vi "Save-Recall Cal Kit.vi"(0 "VISA resource name":refnum<visa-resource-name>, 1 "saver's name":string, 2 "saved cal kit comments":string, 5 "save/load":bool, 7 "file name (read description)":path, 11 "error in (no error)":errorcluster, 12 "saved cal kit title":string) -> (3 "recaller's name":string, 4 "VISA resource name out":refnum<visa-resource-name>, 6 "recalled cal kit comments":string, 8 "recalled cal kit date":string, 10 "recalled cal kit time":string, 14 "recalled cal kit title":string, 15 "error out":errorcluster)   [LabVIEW 2018, in "Agilent 87XX Series.lvlib"]
doc: "This VI for the HP8753B Network Analyzer is used to save and recall modified calibration kit information. The cal kit information is encoded as a form 1 string."
uses:
  Agilent 87XX Series.lvlib
panel:
  # "save to file\nrecall from file"
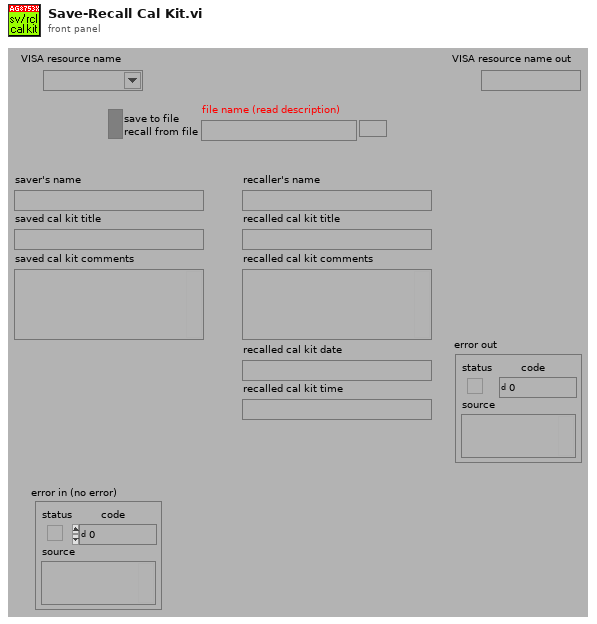
[diagram p1: front panel]
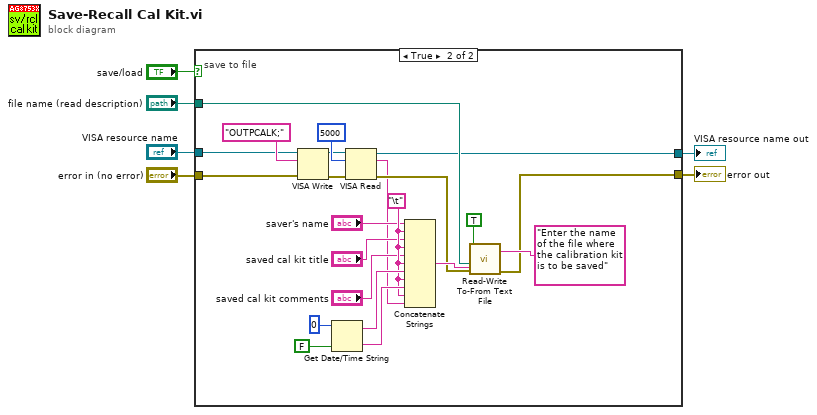
[diagram p0: block diagram]
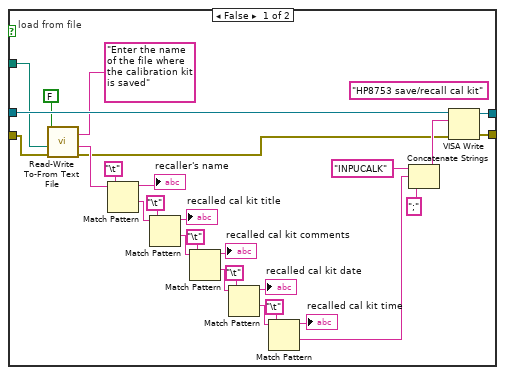
[diagram p2: hidden frame]
diagram:
  n1 = case shown="True" "save/load" {
    tunnel: "file name (read description)" -> [w15 w44]
    tunnel: "VISA resource name" -> [w16 w45]
    tunnel: "error in (no error)" -> [w9 w40]
    tunnel: [w11 w37] -> w2
    tunnel: [w10 w38] -> w1
    frame False {
      (unwired) "HP8753 save/recall cal kit"
      # "load from file"
      n2 = call "Read-Write To-From Text File.vi"("dialog box prompt"="Enter the name of the file where the calibration kit is saved", "error in (no error)"=w9, "file name (read description)"=w15, "read/write (f:read)"=FALSE) -> ("error out"=w8:errorcluster, "string which was read"=w13:string)  [unwired: 6 in]
      n3 = Match Pattern(string=w13, regular expression="\t") -> (before substring=→"recaller's name":string, after substring=w28:string)  [unwired: 1 in, 2 out]
      n4 = Match Pattern(string=w28, regular expression="\t") -> (before substring=→"recalled cal kit title":string, after substring=w27:string)  [unwired: 1 in, 2 out]
      n5 = Match Pattern(string=w27, regular expression="\t") -> (before substring=→"recalled cal kit comments":string, after substring=w23:string)  [unwired: 1 in, 2 out]
      n6 = Match Pattern(string=w23, regular expression="\t") -> (before substring=→"recalled cal kit date":string, after substring=w26:string)  [unwired: 1 in, 2 out]
      n7 = Match Pattern(string=w26, regular expression="\t") -> (before substring=→"recalled cal kit time":string, after substring=w7:string)  [unwired: 1 in, 2 out]
      n8 = Concatenate Strings("INPUCALK", w7, ";") -> (w32:string)
      n9 = VISA Write(VISA resource name=w16, write buffer=w32, error in (no error)=w8) -> (VISA resource name out=w11:refnum<visa-resource-name>, error out=w10:errorcluster)  [unwired: 1 out]
    }
    frame True {
      w49 = "\t"
      # "save to file"
      n10 = VISA Write(VISA resource name=w45, write buffer="OUTPCALK;", error in (no error)=w40) -> (VISA resource name out=w34:refnum<visa-resource-name>, error out=w55:errorcluster)  [unwired: 1 out]
      n11 = Get Date/Time String(date format (0)=0, want seconds? (F)=FALSE) -> (date string=w51:string, time string=w50:string)  [unwired: 1 in]
      n12 = VISA Read(VISA resource name=w34, byte count=u32 5000, error in (no error)=w55) -> (VISA resource name out=w37:refnum<visa-resource-name>, read buffer=w36:string, error out=w39:errorcluster)  [unwired: 1 out]
      n13 = Concatenate Strings("saver's name", w49, "saved cal kit title", w49, "saved cal kit comments", w49, w51, w49, w50, w49, w36) -> (w42:string)
      n14 = call "Read-Write To-From Text File.vi"("string to be written"=w42, "dialog box prompt"="Enter the name of the file where the calibration kit is to be saved", "error in (no error)"=w39, "file name (read description)"=w44, "read/write (f:read)"=TRUE) -> ("error out"=w38:errorcluster)  [unwired: 5 in, 1 out]
    }
  }
  "error out" <- w1
  "VISA resource name out" <- w2
